vi "Turret-firstVI.vi"(0 "Softstop":dbl, 1 "shooter range":dbl=90.0 format="%#_13g", 4 "desired Angle":dbl, 6 "Current angle":dbl, 7 "PID gains":T1={"proportional gain (Kc)"=1.0, "integral time (Ti, min)"=0.01, "derivative time (Td, min)"=0.0} {"derivative time (Td, min)" format="%.3f"; "integral time (Ti, min)" format="%.3f"; "proportional gain (Kc)" format="%.3f"}, 8 "Negative soft stop":bool, 9 "Positive soft stop":bool, 10 "output range":cluster{"output high":dbl, "output low":dbl}={"output high"=1.0, "output low"=-1.0}, 11 "MotorControlDevRef":T2={"DeviceStatus"={"status"=FALSE, "code"=0, "source"=""}, "Type"=enum."PWM", "PWM"={"PWM Channel"=enum."Invalid", "DeadBand"={"Name"="", "maxPositivePwm"=0, "minPositivePwm"=0, "centerPwm"=0, "maxNegativePwm"=0, "minNegativePwm"=0, "angularRange"=0}}, "CAN"={"Device Number"=0, "SetOutput VI Ref"=variant(enum8{"Percent VBus", "Current", "Speed", "Position", "Voltage"} enum."Percent VBus"), "GetOutput VI Ref"=variant(refnum<k1> refnum), "Enable VI Ref"=variant(dbl 12.0), "Disable VI Ref"=variant(enum8{"Percent VBus", "Speed", "Position", "Slave", "Unchanged / Invalid"} enum."Percent VBus"), "Data"=variant}, "Invert"=FALSE}) -> (5 "Motor Output":dbl)   [LabVIEW 2016]
uses:
  <vilib>/Rock Robotics/WPI/MotorControl/WPI_MotorControlDeviceRef.ctl
  <vilib>/Rock Robotics/WPI/MotorControl/WPI_MotorControlType.ctl
  <vilib>/Rock Robotics/SystemInterfaces/DIO/FPGA_DIOPWMChannel.ctl
  <vilib>/Rock Robotics/WPI/PWM/WPI_PWMDeadband.ctl
  <vilib>/addons/control/pid/pid.llb/PID (DBL).vi
  <vilib>/addons/control/pid/NI_PID_pid.lvlib
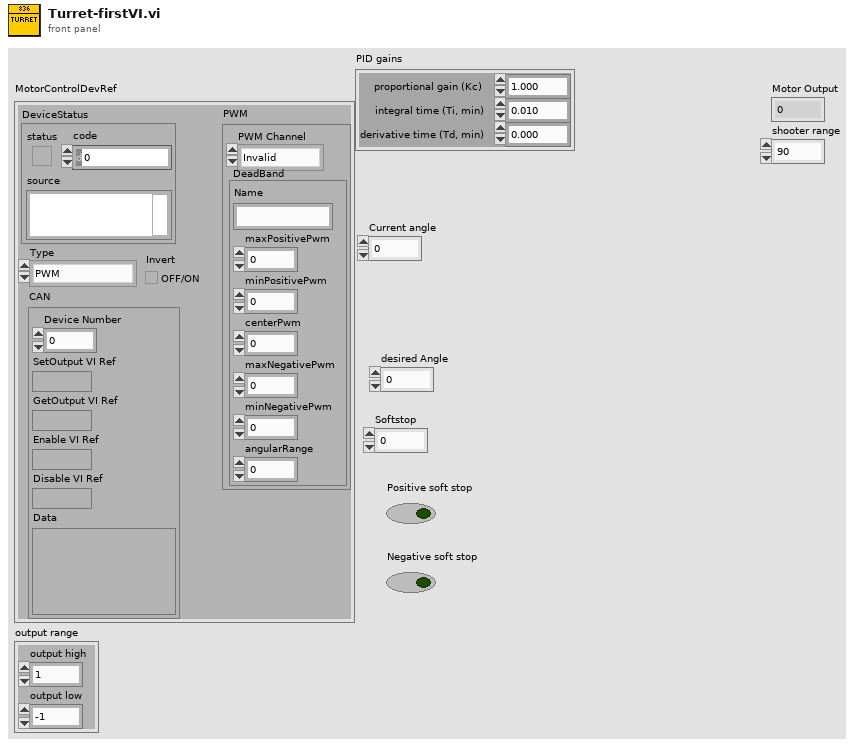
[diagram p1: front panel]
types:
  T1 = cluster{"proportional gain (Kc)":dbl, "integral time (Ti, min)":dbl, "derivative time (Td, min)":dbl}
  T2 = typedef "WPI_MotorControlDeviceRef.ctl" = cluster{"DeviceStatus":errorcluster, "Type":T3, "PWM":cluster{"PWM Channel":T4, "DeadBand":T5}, "CAN":cluster{"Device Number":u8, "SetOutput VI Ref":variant, "GetOutput VI Ref":variant, "Enable VI Ref":variant, "Disable VI Ref":variant, "Data":variant}, "Invert":bool}
  T3 = typedef "WPI_MotorControlType.ctl" = enum16{"PWM", "CAN"}
  T4 = typedef "FPGA_DIOPWMChannel.ctl" = enum8{"PWM 0", "PWM 1", "PWM 2", "PWM 3", "PWM 4", "PWM 5", "PWM 6", "PWM 7", "PWM 8", "PWM 9", "PWM MXP 0", "PWM MXP 1", "PWM MXP 2", "PWM MXP 3", "PWM MXP 4", "PWM MXP 5", "PWM MXP 6", "PWM MXP 7", "PWM MXP 8", "PWM MXP 9", "Invalid"}
  T5 = typedef "WPI_PWMDeadband.ctl" = cluster{"Name":string, "maxPositivePwm":i32, "minPositivePwm":i32, "centerPwm":i32, "maxNegativePwm":i32, "minNegativePwm":i32, "angularRange":u16}
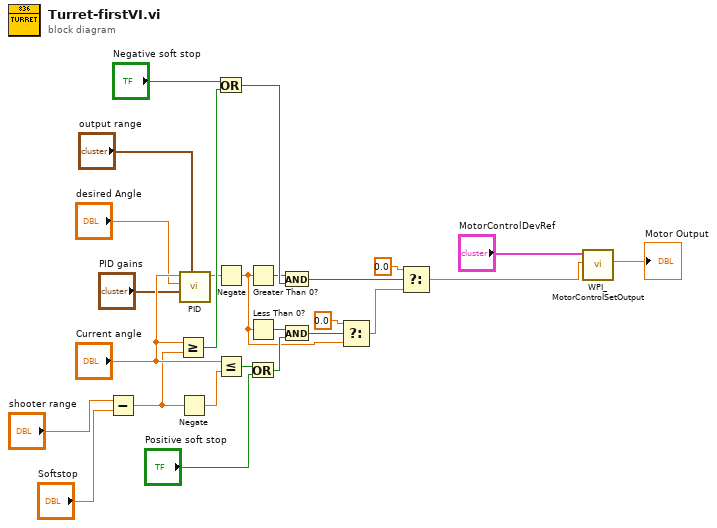
[diagram p0: block diagram]
diagram:
  n1 = Subtract(x="shooter range", y="Softstop") -> (x-y=w5:dbl)
  n2 = Greater Or Equal?(x="Current angle", y=w5) -> (x >= y?=w18:bool)
  n3 = Negate(x=w5) -> (-x=w17:dbl)
  n4 = call-poly <vilib>:"PID.vi"("output range"="output range", "PID gains"="PID gains", "process variable"="desired Angle", "setpoint"="Current angle") -> ("output"=w3:dbl)  [unwired: 6 in, 1 out]
  n5 = Or(x="Negative soft stop", y=w18) -> (x .or. y?=w14:bool)
  n6 = Negate(x=w3) -> (-x=w2:dbl)
  n7 = Less Or Equal?(x="Current angle", y=w17) -> (x <= y?=w21:bool)
  n8 = Greater Than 0?(x=w2) -> (x > 0?=w9:bool)
  n9 = Less Than 0?(x=w2) -> (x < 0?=w10:bool)
  n10 = Or(x=w21, y="Positive soft stop") -> (x .or. y?=w13:bool)
  n11 = And(x=w9, y=w14) -> (x .and. y?=w15:bool)
  n12 = And(x=w10, y=w13) -> (x .and. y?=w16:bool)
  n13 = Select(t=0.0, s=w16, f=w2) -> (s? t:f=w23:dbl)
  n14 = Select(t=0.0, s=w15, f=w23) -> (s? t:f=w22:dbl)
  n15 = call <vilib>:"WPI_MotorControlSetOutput.vi"("Output"=w22, "MotorControlDevRef"="MotorControlDevRef") -> ("Motor Output"=→"Motor Output":dbl)  [unwired: 7 in, 2 out]
